vi "Peak Func.vi"(10 "Y In":dbl[](array[numeric]), 11 "X In":dbl[](array[numeric])) -> (1 "Z":dbl[][](array[numeric]), 2 "Y Out":dbl[](array[numeric]), 3 "X Out":dbl[](array[numeric]))   [LabVIEW 2023]
doc: "Calculate the peak function."
uses:
  <vilib>/gmath/interp.llb/Create Mesh Grid (2D) (x,y arrays).vi
  <vilib>/gmath/NI_Gmath.lvlib
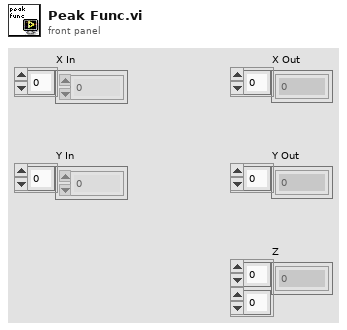
[diagram p1: front panel]
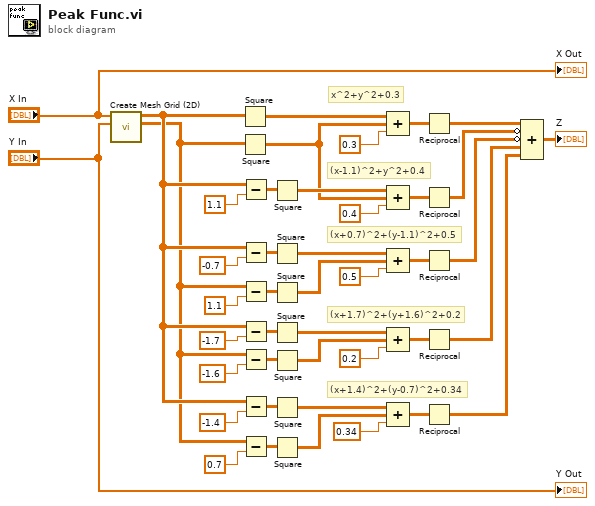
[diagram p0: block diagram]
diagram:
  # "(x+1.4)^2+(y-0.7)^2+0.34"
  # "(x+1.7)^2+(y+1.6)^2+0.2"
  # "(x+0.7)^2+(y-1.1)^2+0.5"
  # "(x-1.1)^2+y^2+0.4"
  # "x^2+y^2+0.3"
  n1 = call-poly <vilib>:"Create Mesh Grid (2D).vi"("y domain"="Y In", "x domain"="X In") -> ("Y"=w1:dbl[][], "X"=w4:dbl[][])  [unwired: 7 in, 1 out]
  n2 = Square(x=w4) -> (x^2=w16:dbl[][])
  n3 = Square(x=w1) -> (x^2=w14:dbl[][])
  n4 = Subtract(x=w4, y=1.1) -> (x-y=w41:dbl[][])
  n5 = Subtract(x=w4, y=-0.7) -> (x-y=w32:dbl[][])
  n6 = Subtract(x=w1, y=1.1) -> (x-y=w31:dbl[][])
  n7 = Subtract(x=w4, y=-1.7) -> (x-y=w27:dbl[][])
  n8 = Subtract(x=w1, y=-1.6) -> (x-y=w29:dbl[][])
  n9 = Subtract(x=w4, y=-1.4) -> (x-y=w20:dbl[][])
  n10 = Subtract(x=w1, y=0.7) -> (x-y=w18:dbl[][])
  n11 = Square(x=w41) -> (x^2=w15:dbl[][])
  n12 = Square(x=w32) -> (x^2=w13:dbl[][])
  n13 = Square(x=w31) -> (x^2=w12:dbl[][])
  n14 = Square(x=w27) -> (x^2=w11:dbl[][])
  n15 = Square(x=w29) -> (x^2=w10:dbl[][])
  n16 = Square(x=w20) -> (x^2=w9:dbl[][])
  n17 = Square(x=w18) -> (x^2=w8:dbl[][])
  n18 = Compound Arithmetic op=ADD(w16, w14, 0.3) -> (w42:dbl[][])
  n19 = Compound Arithmetic op=ADD(w15, w14, 0.4) -> (w38:dbl[][])
  n20 = Compound Arithmetic op=ADD(w13, w12, 0.5) -> (w35:dbl[][])
  n21 = Compound Arithmetic op=ADD(w11, w10, 0.2) -> (w24:dbl[][])
  n22 = Compound Arithmetic op=ADD(w9, w8, 0.34) -> (w22:dbl[][])
  n23 = Reciprocal(x=w42) -> (1/x=w37:dbl[][])
  n24 = Reciprocal(x=w38) -> (1/x=w36:dbl[][])
  n25 = Reciprocal(x=w35) -> (1/x=w30:dbl[][])
  n26 = Reciprocal(x=w24) -> (1/x=w23:dbl[][])
  n27 = Reciprocal(x=w22) -> (1/x=w17:dbl[][])
  n28 = Compound Arithmetic op=ADD(w37, invert w36, invert w30, w23, w17) -> (→"Z":dbl[][])
  "X Out" <- "X In"
  "Y Out" <- "Y In"
